vi "LoadFromINI.vi"(8 "error in (no error)":errorcluster, 10 "path":path, 11 "reference in":refnum<class "niMmWave_Transceiver.lvclass">) -> (0 "error out":errorcluster, 3 "reference out":refnum<class "niMmWave_Transceiver.lvclass">)   [LabVIEW 2019, in "niMmWave_Transceiver.lvclass"]
doc: "Loads insturment data from ini file"
uses:
  niMmWave_Transceiver.lvclass
  <vilib>/Utility/error.llb/Error Cluster From Error Code.vi
  <vilib>/ErrorRing/Error Ring.xnode
  <vilib>/Utility/config.llb/NI_LVConfig.lvlib
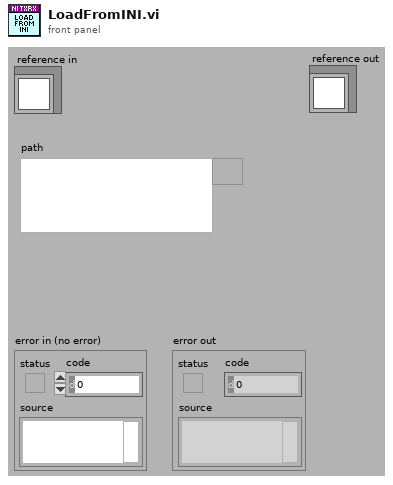
[diagram p1: front panel]
types:
  T1 = cluster{"TX_DAC":string, "TX_FPGA":string, "IF":string, "RX_ADC":string, "RX_FPGA":string}
  T2 = typedef "niMmWave_Transceiver.lvclass/ObjectAttributesRef.ctl" = refnum<data-value>
  T3 = typedef "NI_LVConfig.lvlib/Config Data RefNum.ctl" = refnum<k1>
  T4 = typedef "niMmWave_Transceiver.lvclass/ObjectAttributes.ctl" = cluster{"session":T5[], "HW.RX resources":T19, "RF config":T20, "RX trigger options":T21, "TX trigger options":T21, "RX samples":i32, "Downloaded Bursts":map{string, T24}, "TX Fs":dbl, "RX Fs":dbl, "burst sequence":string[]}
  T5 = typedef "Session.ctl" = cluster{"3620 session":refnum<queue>, "tx baseband session":T6, "rx baseband session":T14, "tx gain (dB)":dbl, "rx gain (dB)":dbl, "hardware configuration":T15, "gain ranging":T17[], "pxi trigger bus information":T18}
  T6 = typedef "Tx Baseband Session.ctl" = cluster{"3610 session":T7, "7902 reference":T13}
  T7 = typedef "ni3610_and_ni3630_Driver_Lib.lvlib/Main Settings.ctl" = cluster{"VISA resource name":refnum<visa-resource-name>, "Address Space":T8, "window_offset":u32, "register_addresses":T9, "required_MM_fpga_version":cluster{"signature":u32, "hardware":u32, "current revision":u32, "oldest revision":u32}, "CPLD Oldest Compat Version ":cluster{"hardware":u32, "CPLD firmware":u32}, "MM_FPGA_image_location":string, "is_init":bool, "card_type":T10, "DacLmkConfigFileName":string, "AdcLmkConfigFileName":string, "AdcConfigFileName":string, "DacConfigFileName_RevA":string, "DacConfigFileName_RevB":string, "Mulde hardware revision":u8, "bypass DAC PLL\n":bool, "IQ Card Revision":T11, "board capability":T12}
  T8 = typedef "VISA Register Access Address Space.ctl" = u16
  T9 = typedef "ni3610_and_ni3630_Driver_Lib.lvlib/Register Adresses.ctl" = cluster{"MM based Registers":cluster{"Revision":u32, "OldestCompatRev":u32, "signature":u32, "scratch":u32, "LedControl":u32, "BoardHwRev":u32, "BoardControl":u32, "ThermalStatus":u32, "BasebandStatus":u32, "BasebandControl":u32, "BasebandAuxSetup":u32, "BasebandAuxStatus":u32, "LmkSyncOutSetup":u32, " AdcSyncOutSetup":u32, " InjSyncOutSetup":u32, " PxiTrig0OutSetup":u32, " PxiTrig1OutSetup":u32, " PxiTrig2OutSetup":u32, " PxiTrig3OutSetup":u32, " PxiTrig4OutSetup":u32, " PxiTrig5OutSetup":u32, " PxiTrig6OutSetup":u32, " PxiTrig7OutSetup":u32}, "CPLD based Registers":cluster{"SlaveSignature":u32, "SlaveRevision":u32, "SlaveOldestCompatRev":u32, "SlaveScratch":u32, "SlaveSetup":u32, "SlaveStatus":u32, "IDacReg_offset":u32, "LMKRegGrp0_offset":u32, "QDacReg_offset":u32, "BrdTempSensorVal":u32, "TempSensorPowerDown":u32, "GPIOReg_offset":u32, "IAdcReg_offset":u32, "QAdcReg_offset":u32, "LMKRegGrp1_offset":u32, "QadcTempSensorVal":u32, "IadcTempSensorVal":u32, "RevisionReg":u32, "VcxoReg":u32, "CpldStatusReg":u32, "PowerReg":u32, "VBiasEnReg":u32, "ExtRefOeReg":u32, "QdacCtrlReg":u32, "QdacStatusReg":u32, "IdacCtrlReg":u32, "IdacStatusReg":u32, "QdacJtagIn":u32, "QdacJtagOut":u32, "IdacJtagIn":u32, "IdacJtagOut":u32, "IqDcSetupReg":u32, "QadcStatusReg":u32, "IadcStatusReg":u32, "BrdSetupReg":u32, "IqDcRevisionReg":u32, "PllStatusReg":u32, "EndpointScratchReg":u32, "AdcSyncCfgReg":u32, "IqCardOpampReg":u32}, "CPLD Register Offset":u32, "MM  Register Offset":u32, " PxiTrig0OutSetup":u32}
  T10 = typedef "ni3610_and_ni3630_Driver_Lib.lvlib/Base Card Type.ctl" = enum16{"unspecified", "ADC", "DAC"}
  T11 = typedef "ni3610_and_ni3630_Driver_Lib.lvlib/IQ Card Revision.ctl" = enum16{"RevA", "RevB", "RevC", "RevD"}
  T12 = typedef "ni3610_and_ni3630_Driver_Lib.lvlib/Board Capability.ctl" = cluster{"baseband sync":enum16{"no baseband sync", "baseband sync"}}
  T13 = typedef "Blank FPGA Reference.ctl" = refnum<k20>
  T14 = typedef "Rx Baseband Session.ctl" = cluster{"3630 session":T7, "7902 reference":T13}
  T15 = typedef "Hardware Configuration.ctl" = cluster{"direction":T16, "baseband only":bool}
  T16 = typedef "Direction.ctl" = enum16{"Transceiver", "Receiver", "Transmitter"}
  T17 = typedef "Gain Ranging.ctl" = cluster{"gain ranging active scope":string, "gain ranging stream session":refnum<k20>}
  T18 = typedef "PXI Trigger Bus Info.ctl" = cluster{"chassis resource name":refnum<visa-resource-name>, "7902R (TX)":i16, "3610 (TX)":i16, "3620 (IF)":i16, "3630 (RX)":i16, "7902R (RX)":i16}
  T19 = typedef "mmWave HW Control.lvlib/HW TXRX resources cluster.ctl" = cluster{"TX_DAC":refnum<visa-resource-name>, "TX_FPGA":tag, "IF":tag, "RX_ADC":refnum<visa-resource-name>, "RX_FPGA":tag}
  T20 = typedef "mmWave HW Control.lvlib/HW TXRX RF config cluster.ctl" = cluster{"TX.Frequency":dbl, "TX.Gain":dbl, "TX.mmWave adapter":string, "RX.Frequency":dbl, "RX.Gain":dbl, "RX.mmWave adapter":string}
  T21 = typedef "TX trigger config.ctl" = cluster{"delay":dbl, "trig source":T22, "PXI src":i32, "export":T23, "PXI dest":i32}
  T22 = typedef "FPGA Utility.lvlib/FPGA driver trigger source.ctl" = enum16{"Use Tclk", "PXI_Trig", "Aurora RX trig"}
  T23 = typedef "FPGA Utility.lvlib/FPGA driver trigger destination.ctl" = enum16{"None", "Source trig", "Synced trig", "Delayed sync"}
  T24 = typedef "niMmWave_Transceiver.lvclass/BurstInfo.ctl" = cluster{"starting addr":u32, "end addr":u32}
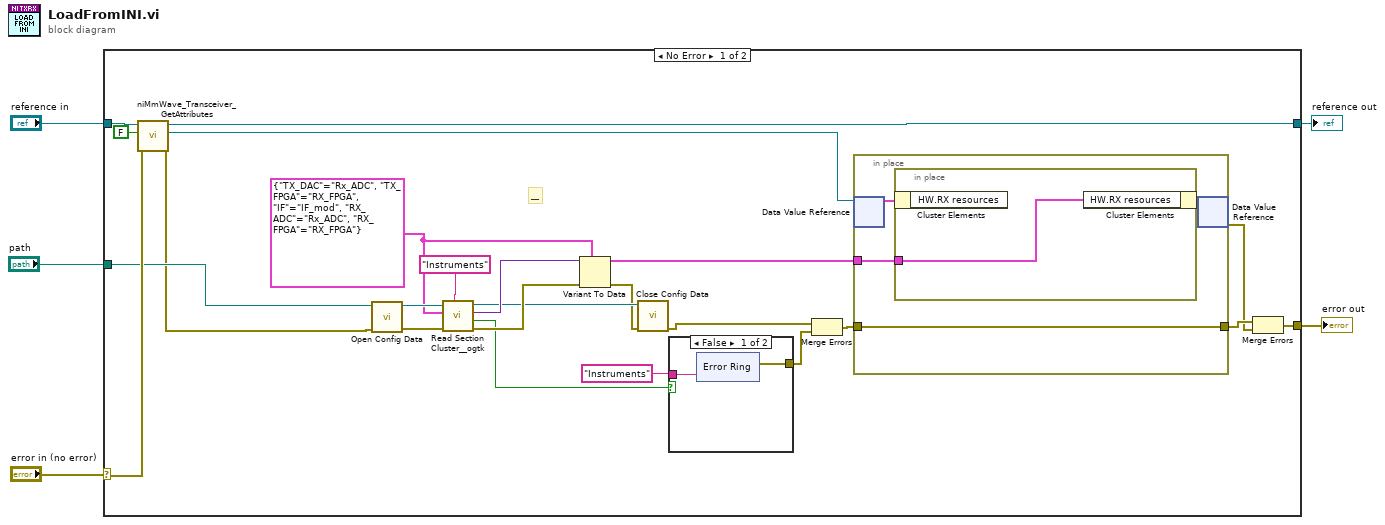
[diagram p0: block diagram]
diagram:
  n1 = case shown="No Error" "error in (no error)" {
    selector: "error in (no error)" -> [w26 w45]
    tunnel: [w29 w45] -> w4
    tunnel: [w27 w44] -> w2
    tunnel: "reference in" -> [w28 w44]
    tunnel: "path" -> [w15 _]
    frame No Error {
      w16 = T1 {"TX_DAC"="Rx_ADC", "TX_FPGA"="RX_FPGA", "IF"="IF_mod", "RX_ADC"="Rx_ADC", "RX_FPGA"="RX_FPGA"} ("HW.RX resources")
      # "__"
      n2 = call "niMmWave_Transceiver_GetAttributes.vi"("error in (no error)"=w26, "return data? (T)"=FALSE, "reference in"=w28) -> ("error out"=w6:errorcluster, "attributes ref"=w23:T2, "reference out"=w27:refnum<class "niMmWave_Transceiver.lvclass">)  [unwired: 5 in, 1 out]
      n3 = call <vilib>:"Open Config Data.vi"("error in (no error)"=w6, "configuration file path"=w15) -> ("error out"=w20:errorcluster, "refnum"=w21:T3)  [unwired: 7 in, 1 out]
      n4 = call <userlib>:"Read Section Cluster__ogtk.vi"("section (optional)"="Instruments", "error in (no error)"=w20, "Section Formatted Cluster Type"=w16, "refnum"=w21) -> ("error out"=w18:errorcluster, "all found?"=w14:bool, "Section Formatted Cluster"=w19:variant, "dup refnum"=w10:T3)  [unwired: 3 in, 1 out]
      n5 = Variant To Data(error in=w18, type=w16, Variant=w19) -> (data=w11:T1, error out=w9:errorcluster)
      n6 = call <vilib>:"Close Config Data.vi"("error in (no error)"=w9, "refnum"=w10) -> ("error out"=w8:errorcluster)  [unwired: 8 in, 1 out]
      n7 = case shown="False" w14 {
        tunnel: "Instruments" ("section (optional)") -> [w36 _]
        tunnel: [w35 _] -> w12
        frame False {
          n8 = xnode "Error Ring"("parameter 0"=w36) -> ("error out"=w35:errorcluster)
        }
        frame True {
        }
      }
      n9 = Merge Errors(w8, w12) -> (w7:errorcluster)
      n10 = in-place {
        in-place-border: w7 -> [w31]
        in-place-border: [w31] -> w25
        in-place-border: w11 -> [w30]
        n11 = in-place-dvr #1(w23) -> (w32:T4)  [unwired: 1 out]
        n12 = in-place {
          in-place-border: w30 -> [w34]
          n13 = in-place-cluster #2(w32) -> ()  [unwired: 1 out]
          n14 = in-place-cluster #2("HW.RX resources"=w34) -> (w33:T4)
        }
        n15 = in-place-dvr #1(w33) -> (w24:errorcluster)  [unwired: 1 out]
      }
      n16 = Merge Errors(w25, w24) -> (w29:errorcluster)
    }
    frame Error {
    }
  }
  "error out" <- w4
  "reference out" <- w2
